vi "PopulateRingArrays.vi"(10 "array":string[](array[string]), 11 "Array Reference":refnum<vi>) -> (0 "error out":errorcluster, 3 "reference out":refnum<vi>)   [LabVIEW 2016]
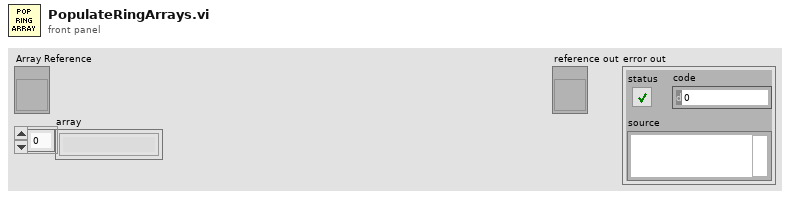
[diagram p1: front panel]
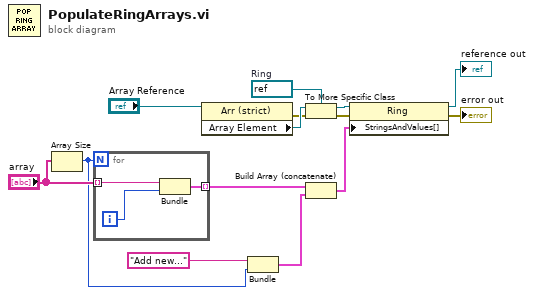
[diagram p0: block diagram]
diagram:
  w13 = refnum<vi> refnum  # Ring
  n1 = Array Size(array="array") -> (size(s)=w1:i32)
  n2 = for {
    N: w1 -> [_]
    tunnel: "array" -> [w17] mode=indexing
    tunnel: [w16] -> w5 mode=indexing
    i -> [w15]
    n3 = Bundle(w17, w15) -> (w16:cluster{string, i32})  [unwired: 1 in]
  }
  n4 = property class="Arr (strict)"(reference="Array Reference") -> (error out=w11:errorcluster, "Array Element"=w14:refnum<vi>)  [unwired: 1 in, 1 out]
  n5 = Bundle("Add new...", w1) -> (w3:cluster{string, i32})  [unwired: 1 in]
  n6 = To More Specific Class(target class=w13, reference=w14, error in=w11) -> (specific class reference=w12:refnum<vi>, error out=w10:errorcluster)
  n7 = Build Array (concatenate)(w5, w3) -> (w2:cluster{string, i32}[])
  n8 = property class="Ring"(reference=w12, error in=w10, "StringsAndValues[]"=w2) -> (reference out=→"reference out":refnum<vi>, error out=→"error out":errorcluster)
